vi "Set Error Messages.vi"(8 "error in":errorcluster, 11 "Errors Node":refnum<k20>) -> (0 "error out":errorcluster, 3 "Errors":T1(array[cluster]))   [LabVIEW 2024, in "Config File Parser.lvlib" / "Channel.lvclass"]
uses:
  Channel.lvclass
  <vilib>/xml/Close Reference(Node).vi
  Channel.lvclass/Channel.ctl
  Config File Parser.lvlib
  <resource>/objmgr/DOMUserDefRef.rc
  <vilib>/xml/NI_XML.lvlib
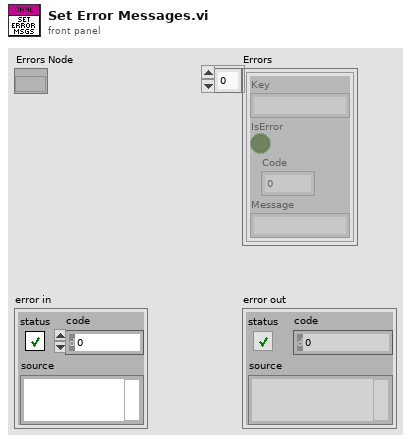
[diagram p1: front panel]
types:
  T1 = cluster{"Key":string, "IsError":bool, "Code":u32, "Message":string}[]
  T2 = cluster{"Key":string, "IsError":bool, "Code":u32, "Message":string}
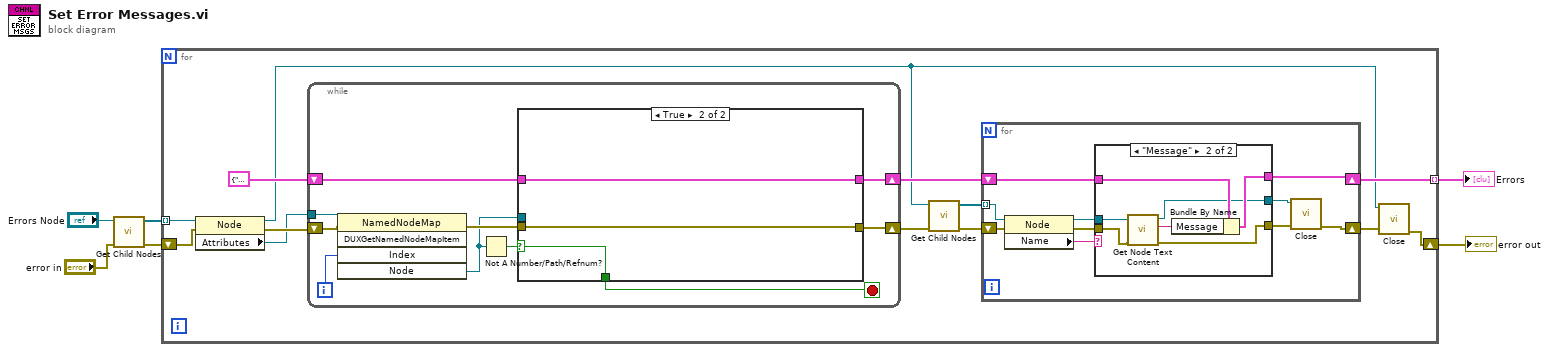
[diagram p0: block diagram]
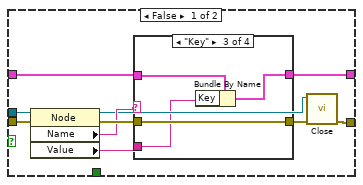
[diagram p2: hidden frame]
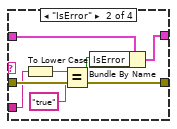
[diagram p4: hidden frame]
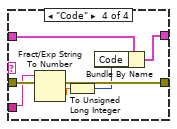
[diagram p5: hidden frame]
diagram:
  n1 = call "Get Child Nodes.vi"("error in"="error in", "Node"="Errors Node") -> ("error out"=w5:errorcluster, "Child Nodes"=w2:refnum<k20>[])  [unwired: 8 in]
  n2 = for {
    tunnel: w2 -> [w10] mode=indexing
    tunnel: [w8] -> w1 mode=indexing
    shift-right: [w14] -> w4
    shift-left: w5 -> [w16]
    n3 = property on="Property Node" class="Node"(reference=w10, error in=w16) -> (reference out=w7:refnum<k20>, error out=w19:errorcluster, "Attributes"=w12:refnum<k20>)
    n4 = while {
      tunnel: w12 -> [w26]
      shift-right: [w27] -> w18
      shift-left: w19 -> [w29]
      shift-right: [w20] -> w11
      shift-left: T2 {"Key"="", "IsError"=FALSE, "Code"=0, "Message"=""} ("Error") -> [w21]
      i -> [w25]
      stop <- w22 stop-if-true
      n5 = invoke on="Invoke Node" class="NamedNodeMap" method="DUXGetNamedNodeMapItem"(reference=w26, error in=w29, "Index"=w25) -> (error out=w28:errorcluster, "Node"=w24:refnum<k20>)  [unwired: 2 in, 3 out]
      n6 = Not A Number/Path/Refnum?(number/path/refnum=w24) -> (NaN/Path/Refnum?=w23:bool)
      n7 = case shown="True" w23 {
        selector: w23 -> [_ w60]
        tunnel: w28 -> [w39 w61]
        tunnel: [w36 w61] -> w27
        tunnel: w24 -> [w35 _]
        tunnel: [_ w60] -> w22
        tunnel: w21 -> [w33 w59]
        tunnel: [w31 w59] -> w20
        frame False {
          n8 = property on="Property Node" class="Node"(reference=w35, error in=w39) -> (reference out=w30:refnum<k20>, error out=w38:errorcluster, "Name"=w34:string, "Value"=w32:string)
          n9 = case shown="\"Key\"" w34 {
            tunnel: w33 -> [w40 w47 w51 w57]
            tunnel: w32 -> [_ w45 w50 w55]
            tunnel: [w40 w46 w49 w56] -> w31
            tunnel: w38 -> [w41 w48 w52 w58]
            tunnel: [w41 w48 w52 w58] -> w37
            frame "-1", Default {
            }
            frame "IsError" {
              n10 = To Lower Case(string=w45) -> (all lower case string=w44:string)
              n11 = Equal?(x=w44, y="true") -> (x = y?=w42:bool)
              n12 = Bundle By Name(cluster=w47, "IsError"=w42) -> (w46:T2)
            }
            frame "Key" {
              n13 = Bundle By Name(cluster=w51, "Key"=w50) -> (w49:T2)
            }
            frame "Code" {
              n14 = Fract/Exp String To Number(string=w55) -> (number=w54:dbl)  [unwired: 3 in, 1 out]
              n15 = To Unsigned Long Integer(number=w54) -> (unsigned 32bit integer=w53:u32)
              n16 = Bundle By Name(cluster=w57, "Code"=w53) -> (w56:T2)
            }
          }
          n17 = call-poly <vilib>:"Close.vi"("error in (no error)"=w37, "node"=w30) -> ("error out"=w36:errorcluster)  [unwired: 7 in]
        }
        frame True {
        }
      }
    }
    n18 = call "Get Child Nodes.vi"("error in"=w18, "Node"=w7) -> ("error out"=w17:errorcluster, "Child Nodes"=w13:refnum<k20>[])  [unwired: 8 in]
    n19 = for {
      tunnel: w13 -> [w67] mode=indexing
      shift-right: [w68] -> w15
      shift-left: w17 -> [w71]
      shift-right: [w63] -> w8
      shift-left: w11 -> [w65]
      n20 = property on="Property Node" class="Node"(reference=w67, error in=w71) -> (reference out=w64:refnum<k20>, error out=w70:errorcluster, "Name"=w66:string)
      n21 = case shown="\"Message\"" w66 {
        tunnel: w65 -> [w73 w79]
        tunnel: w64 -> [w72 w78]
        tunnel: [w73 w76] -> w63
        tunnel: w70 -> [w74 w81]
        tunnel: [w74 w80] -> w69
        tunnel: [w72 w75] -> w62
        frame "-1", Default {
        }
        frame "Message" {
          n22 = call <vilib>:"Get Node Text Content.vi"("error in (no error)"=w81, "node in"=w78) -> ("error out"=w80:errorcluster, "node text"=w77:string, "node out"=w75:refnum<k20>)  [unwired: 7 in]
          n23 = Bundle By Name(cluster=w79, "Message"=w77) -> (w76:T2)
        }
      }
      n24 = call-poly <vilib>:"Close.vi"("error in (no error)"=w69, "node"=w62) -> ("error out"=w68:errorcluster)  [unwired: 7 in]
    }
    n25 = call-poly <vilib>:"Close.vi"("error in (no error)"=w15, "node"=w7) -> ("error out"=w14:errorcluster)  [unwired: 7 in]
  }
  "Errors" <- w1
  "error out" <- w4
